vi "onProcessStartedWithErrors.vi"(8 "error in (no error)":errorcluster, 10 "Start error":errorcluster, 11 "DAQmx(AI)":refnum<class "DAQmx(AI).lvclass">) -> (0 "error out":errorcluster, 3 "DAQmx(AI) out":refnum<class "DAQmx(AI).lvclass">)   [LabVIEW 2019, in "DAQmx(AI).lvclass"]
doc: "JKI State Machine Objects (SMO) 1.1.8.32\nJKI - JKI\nCopyright (c) 2016, JKI"
uses:
  DAQmx(AI).lvclass
  vi.lib/JKI/JKI SMO/SMO/SMO.lvclass
panel:
  out "Unhandled error":errorcluster
  # "For instructions on how to use the JKI State Machine Objects, examples and video tutorials, visit:\nhttp://jki.net/state-machine-objects/\n\nJKI State Machine Objects™\nhttp://jki.net/state-machine-objects/\nCopyright (C) 2005-2015, JKI <info@jki.net>\nALL RIGHTS RESERVED"
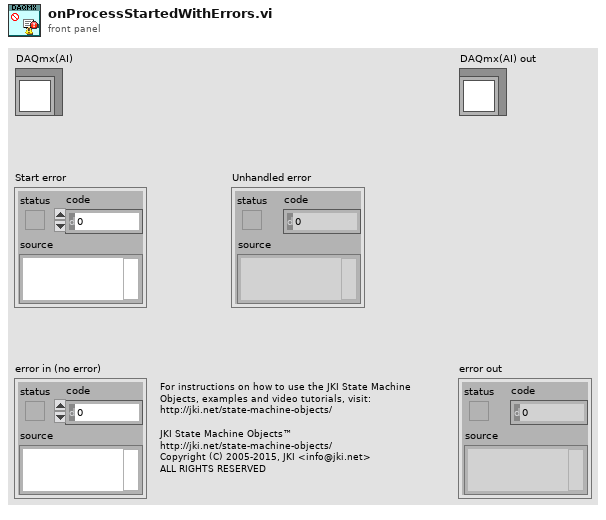
[diagram p1: front panel]
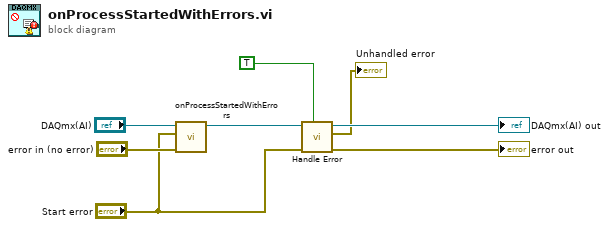
[diagram p0: block diagram]
diagram:
  n1 = call-parent "onProcessStartedWithErrors.vi"("error in (no error)"="error in (no error)", "Start error"="Start error", "SMO"="DAQmx(AI)") -> ("SMO out"=w5:refnum<class "DAQmx(AI).lvclass">)  [unwired: 7 in, 1 out]
  n2 = call-dynamic "Handle Error.vi"("Stop on Unhandled Error (T)"=TRUE, "error in"="Start error", "SMO"=w5) -> ("handling error"=→"error out":errorcluster, "Unhandled error"=→"Unhandled error":errorcluster, "SMO out"=→"DAQmx(AI) out":refnum<class "DAQmx(AI).lvclass">)  [unwired: 6 in]
